vi "Publish Message.vi"(0 "SystemLinkOutputTerminal in":refnum<class "SystemLinkOutputTerminal.lvclass">, 5 "Publish Message":string, 11 "error in (no error)":errorcluster) -> (4 "SystemLinkOutputTerminal out":refnum<class "SystemLinkOutputTerminal.lvclass">, 15 "error out":errorcluster)   [LabVIEW 2016, in "SystemLinkOutputTerminal.lvclass"]
uses:
  SystemLinkOutputTerminal.lvclass
  SystemLinkOutputTerminal.lvclass/SystemLinkOutputTerminal.ctl
  <vilib>/Skyline/Message/AMQP/NI Skyline Message AMQP (Async).lvclass
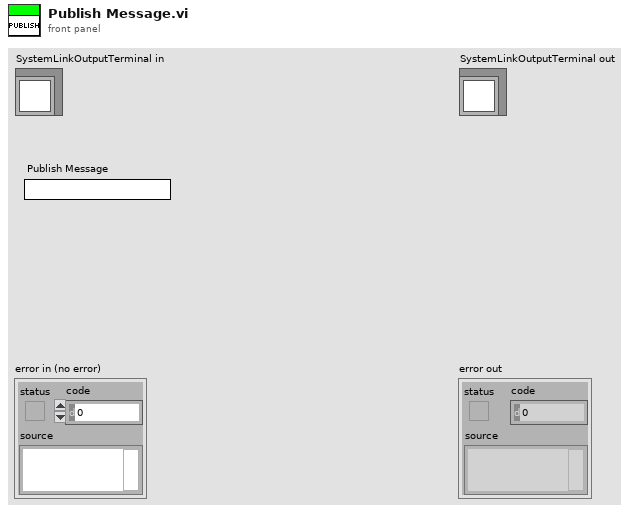
[diagram p1: front panel]
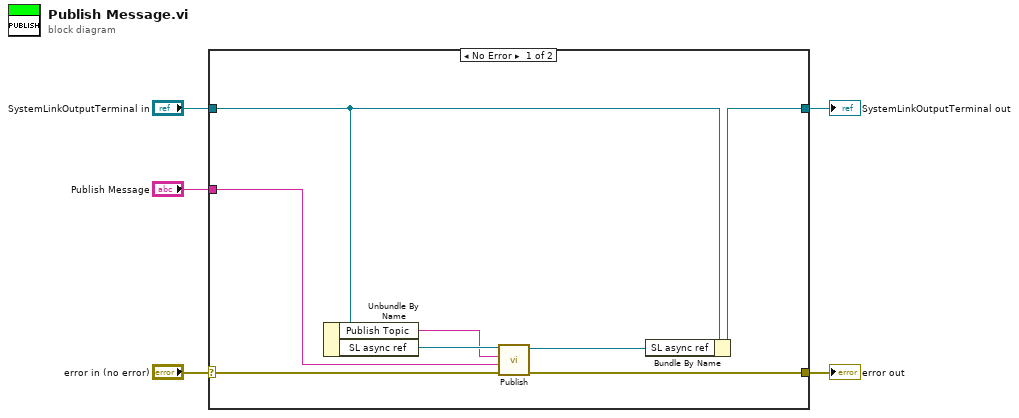
[diagram p0: block diagram]
diagram:
  n1 = case shown="No Error" "error in (no error)" {
    selector: "error in (no error)" -> [w13 w15]
    tunnel: [w12 w15] -> w4
    tunnel: [w8 w14] -> w2
    tunnel: "SystemLinkOutputTerminal in" -> [w9 w14]
    tunnel: "Publish Message" -> [w6 _]
    frame No Error {
      n2 = Unbundle By Name(w9) -> ("Publish Topic"=w7:string, "SL async ref"=w11:refnum<class "NI Skyline Message AMQP (Async).lvclass">)
      n3 = call-dynamic "Publish.vi"("error in (no error)"=w13, "message"=w6, "topic"=w7, "message async"=w11) -> ("error out"=w12:errorcluster, "message async out"=w10:refnum<class "NI Skyline Message AMQP (Async).lvclass">)  [unwired: 6 in]
      n4 = Bundle By Name(cluster=w9, "SL async ref"=w10) -> (w8:refnum<class "SystemLinkOutputTerminal.lvclass">)
    }
    frame Error {
    }
  }
  "error out" <- w4
  "SystemLinkOutputTerminal out" <- w2
